vi "Err Promise Already Resolved.vi"() -> (0 "Error":errorcluster)   [LabVIEW 2017, in "Futures.lvlib" / "Promise.lvclass"]
uses:
  Promise.lvclass
  <vilib>/Utility/error.llb/Error Cluster From Error Code.vi
  <vilib>/ErrorRing/Error Ring.xnode
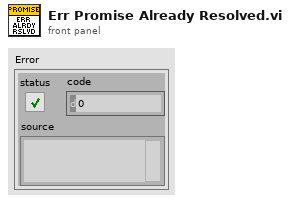
[diagram p1: front panel]
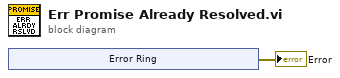
[diagram p0: block diagram]
diagram:
  n1 = xnode "Error Ring"() -> ("error out"=→"Error":errorcluster)
